vi "Teleop.vi"(10 "Match Info":T1={"Autonomous Elapsed Seconds"=0.0, "TeleOp Elapsed Seconds"=0.0, "Disabled Elapsed Seconds"=0.0, "Visited Autonomous"=FALSE, "Visited TeleOp"=FALSE, "Visited Disabled"=FALSE, "Autonomous Settings"={"Autonomous Style"=enum."Independent", "VI Refnum"=refnum}}, 11 "Call Context":T2) -> ()   [LabVIEW 2023]
doc: "This VI is called for each enabled TeleOp packet received from the DS. It is typically used to read from joysticks and other inputs and update I/O or setpoints for timed control loops. It should complete and return within 20 milliseconds or risk missing DS packets."
uses:
  <vilib>/Rock Robotics/WPI/DriverStation/WPI_DriverStationDerivedRobotMode.ctl
  <vilib>/Rock Robotics/WPI/DriverStation/WPI_DriverStationMatch Info.ctl
  <vilib>/Rock Robotics/WPI/Utilities/WPI_GetSetVariantRefNum.vi
  <vilib>/Rock Robotics/Network Tables/NT Write Boolean Array.vi
  <vilib>/Rock Robotics/Network Tables/NT Write Numeric Array.vi
  <vilib>/Rock Robotics/Network Tables/NT Read Number.vi
  MHZLib/Variables and Definitions/Robot Global Data.vi
  <vilib>/Rock Robotics/Network Tables/NT Write Boolean.vi
panel:
  out "Lift dband":dbl
  in  "Lift Lock":bool=TRUE
  out "Drive dband":dbl
  out "Steer dband":dbl
  out "Sprint Mode":bool
  out "Sprint Button":bool
  out "Sprint Throttle":dbl
  out "Drive Throttle":dbl
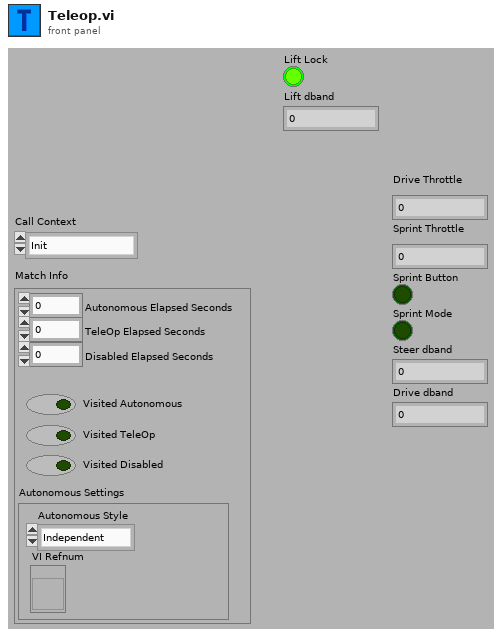
[diagram p1: front panel]
types:
  T1 = typedef "WPI_DriverStationMatch Info.ctl" = cluster{"Autonomous Elapsed Seconds":dbl, "TeleOp Elapsed Seconds":dbl, "Disabled Elapsed Seconds":dbl, "Visited Autonomous":bool, "Visited TeleOp":bool, "Visited Disabled":bool, "Autonomous Settings":cluster{"Autonomous Style":enum16{"Iterative", "Independent"}, "VI Refnum":refnum<vi>}}
  T2 = typedef "WPI_DriverStationDerivedRobotMode.ctl" = enum16{"Init", "Execute", "Stop"}
  T3 = typedef "Auto_Values.ctl" = cluster{"X Pos":dbl, "Y Pos":dbl, "Heading (Deg)":dbl, "Strafe Throttle":dbl, "Rot Throtle (Rad/s)":dbl, "Strafe Tol (Ft)":dbl, "Rotation Tol (Deg)":dbl, "Shooter Pos":enum16{"Hold", "Travel", "Speaker", "Amp"}, "Intake":enum16{"Off", "Front", "Center", "Out"}, "Auto Aim":enum16{"Off", "Aim", "Aim & Shoot"}, "Shooter Throttle":dbl, "Wait (s)":dbl, "Lift":enum16{"Off", "Up", "Down"}, "Shoot?":bool}
  T4 = typedef "WPI_JoystickDevRef.ctl" = cluster{"Device":T5}
  T5 = typedef "WPI_JoystickDeviceEnum.ctl" = enum16{"USB 0", "USB 1", "USB 2", "USB 3", "USB 4", "USB 5"}
  T6 = typedef "WPI_Joystick Info.ctl" = cluster{"Device Name":string, "HID Type":T7, "XBox Type":T8, "Axes Count":i32, "Axes Types":T9[], "Button Count":i32, "POV Count":i32}
  T7 = typedef "WPI_JoystickHID Types.ctl" = enum16{"Not HID", "HID Joystick", "HID Gamepad", "HID Driving Wheel", "HID Flightstick", "HID First Person"}
  T8 = typedef "WPI_JoystickXBox Types.ctl" = enum16{"Not XBox", "XBox Unknown", "XBox Gamepad", "XBox Wheel", "XBox Arcade Stick", "XBox Flight Stick", "XBox Dance Pad", "XBox Guitar", "XBox Drum Kit", "XBox Arcade Pad"}
  T9 = typedef "WPI_JoystickAxis Types.ctl" = enum16{"X Axis", "Y Axis", "Z Axis", "RxAxis", "RyAxis", "RzAxis", "Slider", "POV", "None", "L X Axis", "L Y Axis", "L Trigger", "R Trigger", "R X Axis", "R Y Axis"}
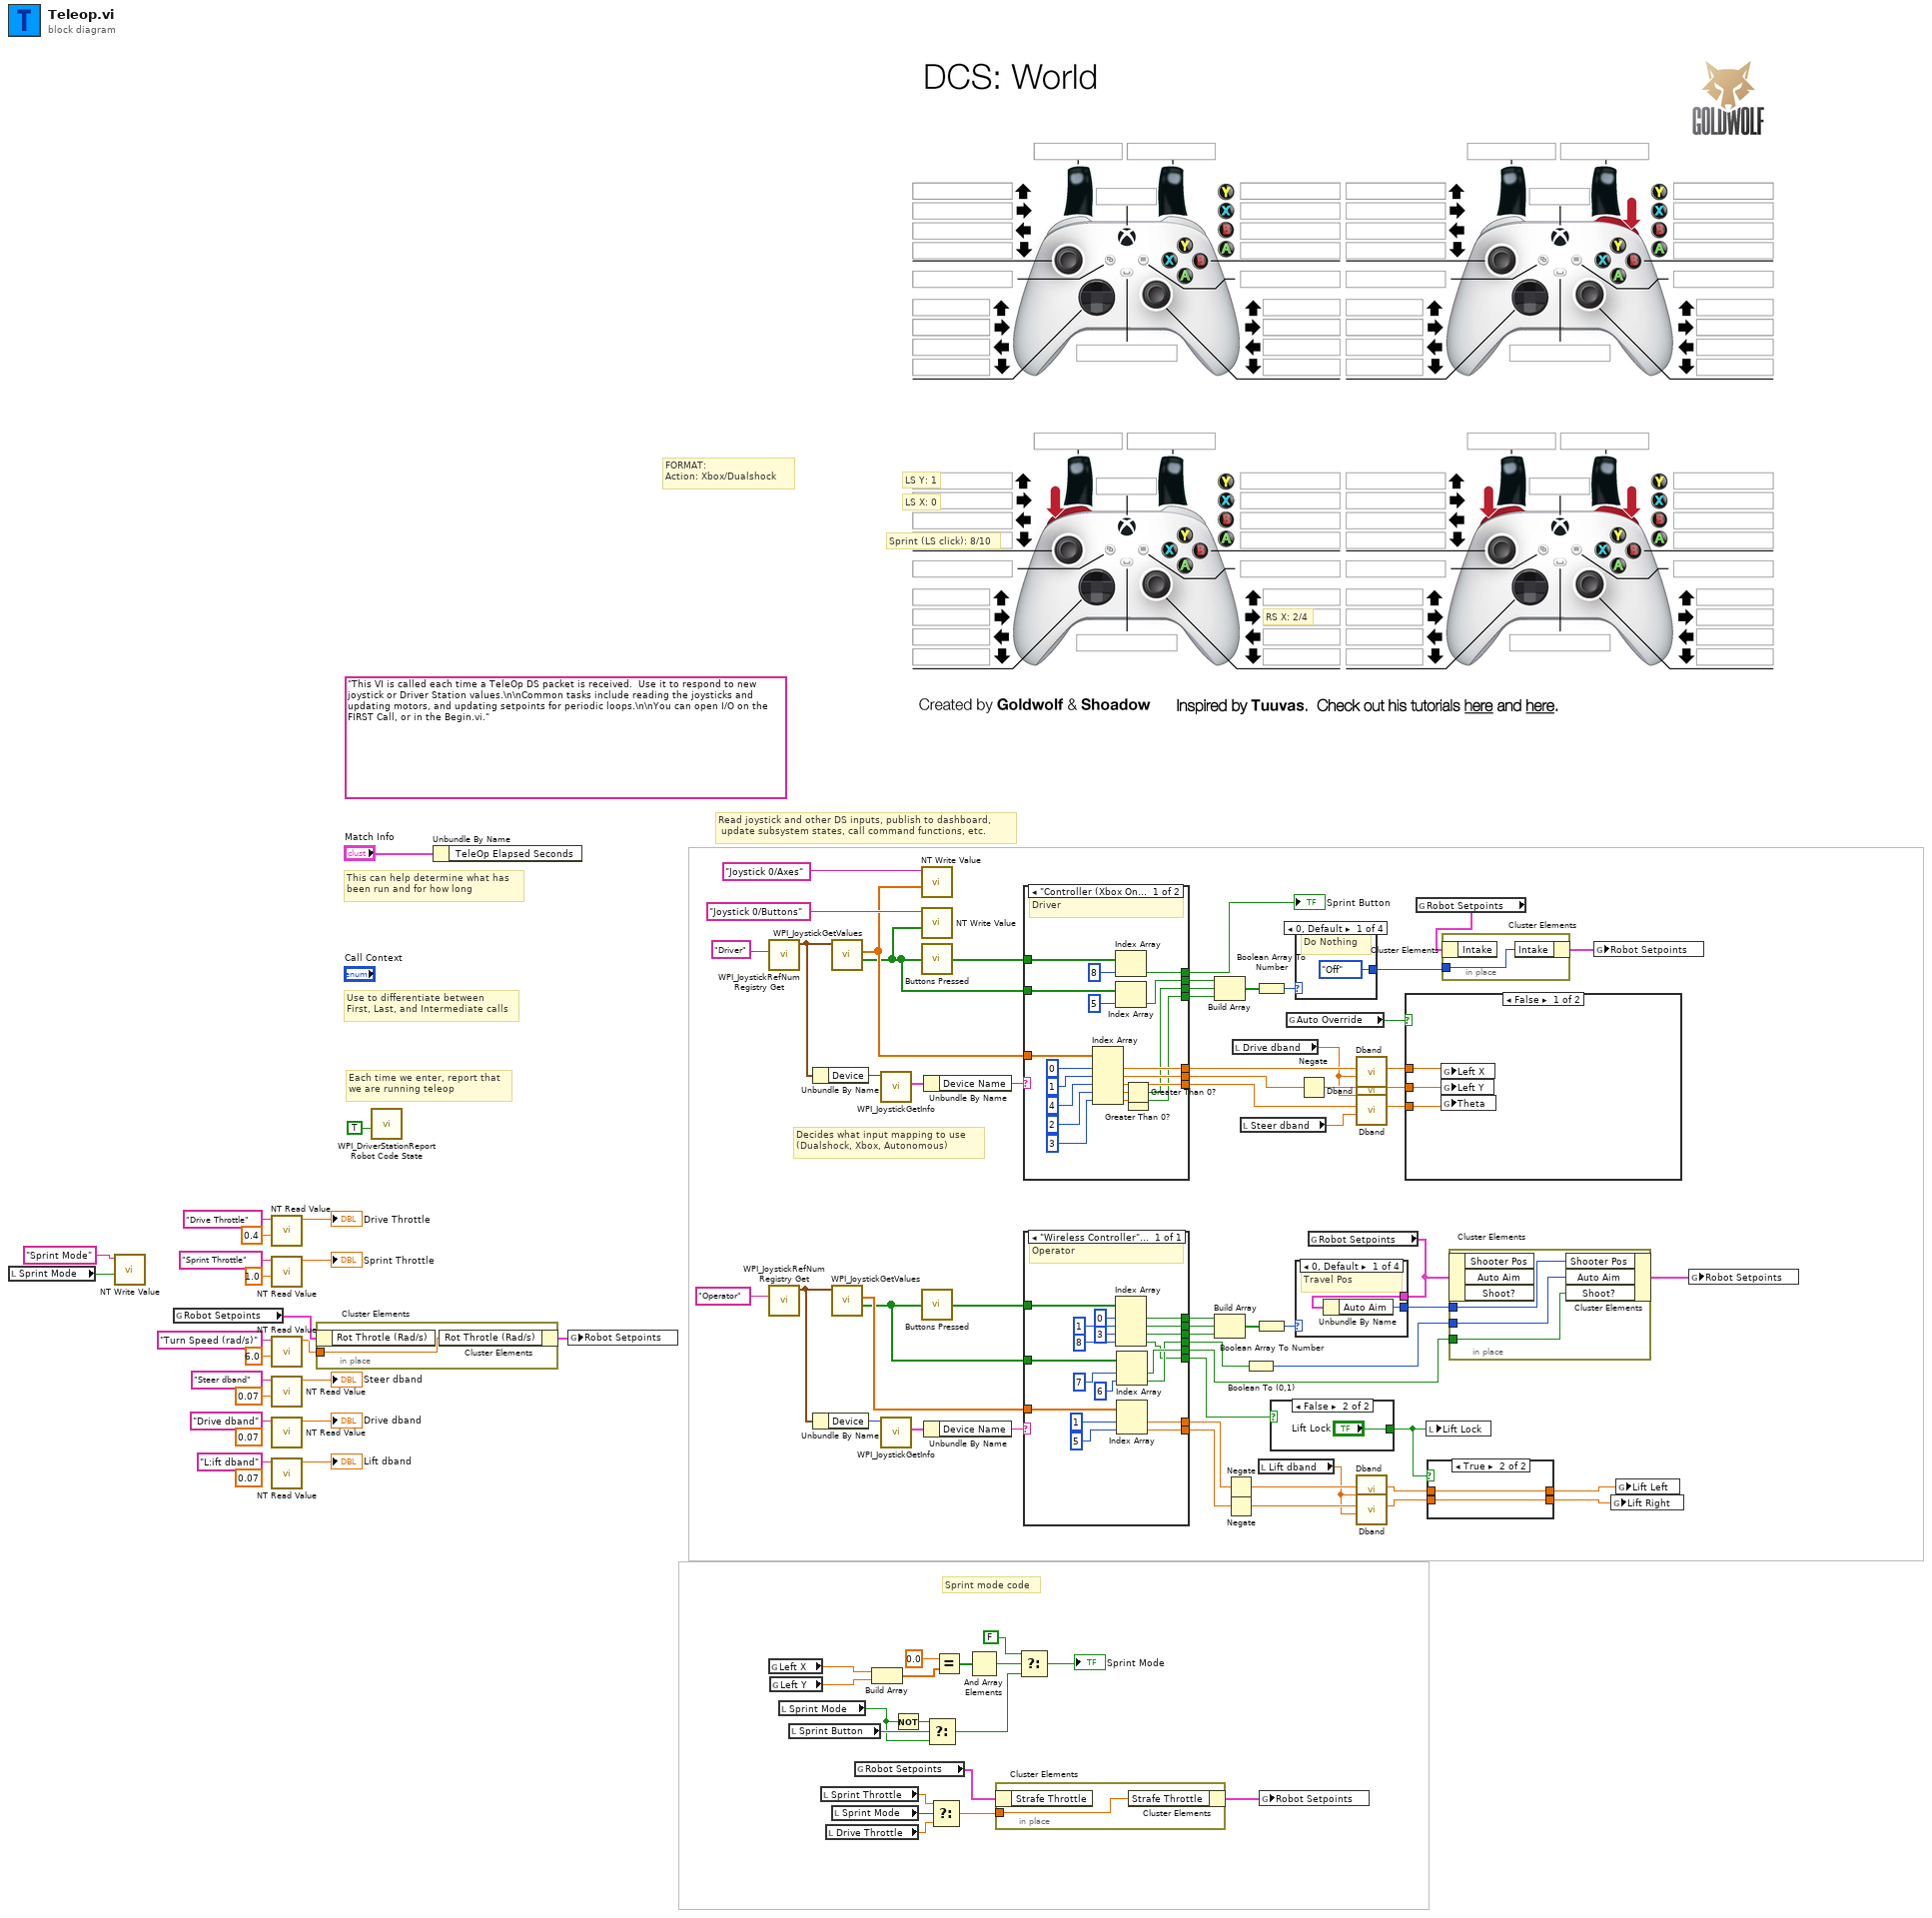
[diagram p0: block diagram]
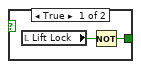
[diagram p2: hidden frame]
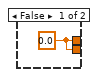
[diagram p3: hidden frame]
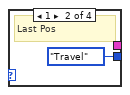
[diagram p4: hidden frame]
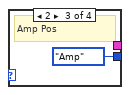
[diagram p5: hidden frame]
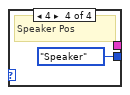
[diagram p6: hidden frame]
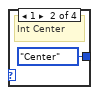
[diagram p7: hidden frame]
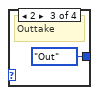
[diagram p8: hidden frame]
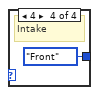
[diagram p9: hidden frame]
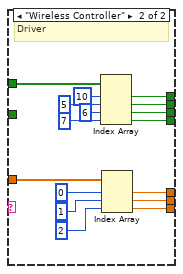
[diagram p11: hidden frame]
diagram:
  (unwired) 0.07 ("default value")
  (unwired) 0.07 ("default value")
  (unwired) "This VI is called each time a TeleOp DS packet is received.  Use it to respond to new joystick or Driver Station values.\n\nCommon tasks include reading the joysticks and updating motors, and updating setpoints for periodic loops.\n\nYou can open I/O on the FIRST Call, or in the Begin.vi."
  # "Sprint mode code"
  # "RS X: 2/4"
  # "LS X: 0"
  # "LS Y: 1"
  # "FORMAT:\nAction: Xbox/Dualshock"
  # "Sprint (LS click): 8/10"
  # "Decides what input mapping to use\n(Dualshock, Xbox, Autonomous)"
  # "Read joystick and other DS inputs, publish to dashboard,\n update subsystem states, call command functions, etc."
  # "Each time we enter, report that\nwe are running teleop"
  # "Use to differentiate between\nFirst, Last, and Intermediate calls"
  # "This can help determine what has\nbeen run and for how long"
  n1 = local read "Sprint Mode"() -> (w50:bool)
  n2 = call-poly <vilib>:"NT Write Value.vi"("value"=w50, "name"="Sprint Mode") -> ()  [unwired: 9 in, 1 out]
  n3 = global read "Robot Global Data.vi" "Robot Setpoints"() -> (w5:T3)
  n4 = call-poly <vilib>:"NT Read Value.vi"("default value"=0.4, "name"="Drive Throttle") -> ("value"=→"Drive Throttle":dbl)  [unwired: 7 in, 2 out]
  n5 = call-poly <vilib>:"NT Read Value.vi"("default value"=1.0, "name"="Sprint Throttle") -> ("value"=→"Sprint Throttle":dbl)  [unwired: 7 in, 2 out]
  n6 = call-poly <vilib>:"NT Read Value.vi"("default value"=6.0, "name"="Turn Speed (rad/s)") -> ("value"=w4:dbl)  [unwired: 7 in, 2 out]
  n7 = call-poly <vilib>:"NT Read Value.vi"("default value"=0.07, "name"="Steer dband") -> ("value"=→"Steer dband":dbl)  [unwired: 7 in, 2 out]
  n8 = call-poly <vilib>:"NT Read Value.vi"("name"="Drive dband") -> ("value"=→"Drive dband":dbl)  [unwired: 8 in, 2 out]
  n9 = call-poly <vilib>:"NT Read Value.vi"("name"="L:ift dband") -> ("value"=→"Lift dband":dbl)  [unwired: 8 in, 2 out]
  n10 = in-place {
    in-place-border: w4 -> [w100]
    n11 = in-place-cluster #1(w5) -> ()  [unwired: 1 out]
    n12 = in-place-cluster #1("Rot Throtle (Rad/s)"=w100) -> (w6:T3)
  }
  n13 = call <vilib>:"WPI_DriverStationReport Robot Code State.vi"("TeleOp"=TRUE ("Autonomous")) -> ()  [unwired: 10 in, 1 out]
  n14 = Unbundle By Name("Match Info") -> ()  [unwired: 1 out]
  n15 = global write "Robot Global Data.vi" "Robot Setpoints"(w6) -> ()
  n16 = call <vilib>:"WPI_JoystickRefNum Registry Get.vi"("refnum name"="Driver") -> ("JoystickDevRef"=w53:T4)  [unwired: 1 in, 9 out]
  n17 = call <vilib>:"WPI_JoystickRefNum Registry Get.vi"("refnum name"="Operator") -> ("JoystickDevRef"=w44:T4)  [unwired: 1 in, 9 out]
  n18 = global read "Robot Global Data.vi" "Left X"() -> (w63:dbl)
  n19 = global read "Robot Global Data.vi" "Left Y"() -> (w62:dbl)
  n20 = local read "Sprint Mode"() -> (w78:bool)
  n21 = local read "Sprint Button"() -> (w79:bool)
  n22 = Unbundle By Name(w53) -> ("Device"=w85:T5)
  n23 = Unbundle By Name(w44) -> ("Device"=w47:T5)
  n24 = local read "Sprint Throttle"() -> (w55:dbl)
  n25 = local read "Drive Throttle"() -> (w54:dbl)
  n26 = call <vilib>:"WPI_JoystickGetValues.vi"("JoystickDevRef"=w53) -> ("Buttons"=w2:bool[], "Axes"=w84:dbl[])  [unwired: 6 in, 3 out]
  n27 = call <vilib>:"WPI_JoystickGetValues.vi"("JoystickDevRef"=w44) -> ("Buttons"=w3:bool[], "Axes"=w43:dbl[])  [unwired: 6 in, 3 out]
  n28 = local read "Sprint Mode"() -> (w56:bool)
  n29 = global read "Robot Global Data.vi" "Robot Setpoints"() -> (w12:T3)
  n30 = Build Array(w63, w62) -> (w60:dbl[])
  n31 = call <vilib>:"WPI_JoystickGetInfo.vi"("JoystickDevice"=w85) -> ("Joystick Info"=w86:T6)  [unwired: 9 in, 1 out]
  n32 = call <vilib>:"WPI_JoystickGetInfo.vi"("JoystickDevice"=w47) -> ("Joystick Info"=w46:T6)  [unwired: 9 in, 1 out]
  n33 = Not(x=w78) -> (.not. x?=w80:bool)
  n34 = call-poly <vilib>:"NT Write Value.vi"("value"=w84, "name"="Joystick 0/Axes" ("Name")) -> ()  [unwired: 9 in, 1 out]
  n35 = call-poly <vilib>:"NT Write Value.vi"("value"=w2, "name"="Joystick 0/Buttons" ("Name")) -> ()  [unwired: 9 in, 1 out]
  n36 = call "Buttons Pressed.vi"("Button Values"=w2) -> ("Button Presses"=w82:bool[])
  n37 = call "Buttons Pressed.vi"("Button Values"=w3) -> ("Button Presses"=w42:bool[])
  n38 = Unbundle By Name(w86) -> ("Device Name"=w83:string)
  n39 = Unbundle By Name(w46) -> ("Device Name"=w45:string)
  n40 = Select(t=w80, s=w79, f=w78) -> (s? t:f=w52:bool)
  n41 = Select(t=w55, s=w56, f=w54) -> (s? t:f=w11:dbl)
  n42 = Equal?(x=0.0, y=w60) -> (x = y?=w59:bool[])
  n43 = And Array Elements(Boolean array=w59) -> (logical AND=w58:bool)
  n44 = in-place {
    in-place-border: w11 -> [w101]
    n45 = in-place-cluster #2(w12) -> ()  [unwired: 1 out]
    n46 = in-place-cluster #2("Strafe Throttle"=w101) -> (w10:T3)
  }
  n47 = Select(t=FALSE, s=w58, f=w52) -> (s? t:f=→"Sprint Mode":bool)
  n48 = case shown="\"Controller (Xbox One For Windows)\", Default" w83 {
    tunnel: w84 -> [w117 w133]
    tunnel: w82 -> [w115 w132]
    tunnel: [w114 w130] -> w81
    tunnel: [w113 w129] -> w68
    tunnel: [w112 w128] -> w67
    tunnel: [w111 w127] -> w66
    tunnel: [w104 w125] -> w40
    tunnel: [w106 w123] -> w39
    tunnel: [w105 w124] -> w38
    tunnel: w2 -> [w102 _]
    frame "Controller (Xbox One For Windows)", Default {
      # "Driver"
      n49 = Index Array(array=w117, index #1=0 ("index"), index #2=1 ("index"), index #3=4 ("index"), index #4=2 ("index"), index #5=3 ("index")) -> (element #1=w113:dbl, element #2=w112:dbl, element #3=w111:dbl, element #4=w108:dbl, element #5=w107:dbl)
      n50 = Index Array(array=w115, index=8) -> (element=w114:bool)
      n51 = Index Array(array=w102, index=5) -> (element=w104:bool)
      n52 = Greater Than 0?(x=w108) -> (x > 0?=w106:bool)
      n53 = Greater Than 0?(x=w107) -> (x > 0?=w105:bool)
    }
    frame "Wireless Controller" {
      # "Driver"
      n54 = Index Array(array=w132, index #1=10 ("index"), index #2=5 ("index"), index #3=6 ("index"), index #4=7 ("index")) -> (element #1=w130:bool, element #2=w125:bool, element #3=w123:bool, element #4=w124:bool)
      n55 = Index Array(array=w133, index #1=0 ("index"), index #2=1 ("index"), index #3=2 ("index")) -> (element #1=w129:dbl, element #2=w128:dbl, element #3=w127:dbl)
    }
  }
  "Sprint Button" <- w81
  n56 = case shown="\"Wireless Controller\", Default" w45 {
    tunnel: w43 -> [w153]
    tunnel: w42 -> [w152]
    tunnel: [w150] -> w35
    tunnel: [w149] -> w25
    tunnel: [w148] -> w26
    tunnel: [w146] -> w34
    tunnel: [w144] -> w33
    tunnel: [w138] -> w29
    tunnel: [w139] -> w27
    tunnel: [w137] -> w22
    tunnel: w3 -> [w140]
    frame "Wireless Controller", Default {
      # "Operator"
      n57 = Index Array(array=w152, index #1=0 ("index"), index #2=1 ("index"), index #3=3 ("index"), index #4=8 ("index")) -> (element #1=w150:bool, element #2=w146:bool, element #3=w144:bool, element #4=w137:bool)
      n58 = Index Array(array=w140, index #1=7 ("index"), index #2=6 ("index")) -> (element #1=w139:bool, element #2=w138:bool)
      n59 = Index Array(array=w153, index #1=1 ("index"), index #2=5 ("index")) -> (element #1=w149:dbl, element #2=w148:dbl)
    }
  }
  n60 = Build Array(w40, w39, w38) -> (w37:bool[])
  n61 = Build Array(w35, w34, w33) -> (w32:bool[])
  n62 = Negate(x=w25) -> (-x=w20:dbl)
  n63 = Negate(x=w26) -> (-x=w19:dbl)
  n64 = local read "Drive dband"() -> (w65:dbl)
  n65 = local read "Steer dband"() -> (w64:dbl)
  n66 = Boolean To (0,1)(Boolean=w29) -> (0, 1=w28:i16)
  n67 = Boolean Array To Number(Boolean array=w37) -> (number=w36:u32)
  n68 = Boolean Array To Number(Boolean array=w32) -> (number=w31:u32)
  n69 = local read "Lift dband"() -> (w16:dbl)
  n70 = global write "Robot Global Data.vi" "Robot Setpoints"(w10) -> ()
  n71 = case shown="False" w22 {
    tunnel: [w156 "Lift Lock"] -> w21
    frame True {
      n72 = local read "Lift Lock"() -> (w157:bool)
      n73 = Not(x=w157) -> (.not. x?=w156:bool)
    }
    frame False {
    }
  }
  n74 = global read "Robot Global Data.vi" "Auto Override"() -> (w48:bool)
  n75 = case shown="0, Default" w36 {
    tunnel: [enum16{"Off", "Front", "Center", "Out"}."Off" ("Intake") enum16{"Off", "Front", "Center", "Out"}."Center" ("Intake") enum16{"Off", "Front", "Center", "Out"}."Out" ("Intake") enum16{"Off", "Front", "Center", "Out"}."Front" ("Intake")] -> w8
    frame 0, Default {
      # "Do Nothing"
    }
    frame 1 {
      # "Int Center"
    }
    frame 2 {
      # "Outtake"
    }
    frame 4 {
      # "Intake"
    }
  }
  n76 = Negate(x=w67) -> (-x=w72:dbl)
  n77 = global read "Robot Global Data.vi" "Robot Setpoints"() -> (w1:T3)
  n78 = case shown="0, Default" w31 {
    tunnel: [w163 enum16{"Hold", "Travel", "Speaker", "Amp"}."Travel" ("Shooter Pos") enum16{"Hold", "Travel", "Speaker", "Amp"}."Amp" ("Shooter Pos") enum16{"Hold", "Travel", "Speaker", "Amp"}."Speaker" ("Shooter Pos")] -> w30
    tunnel: w1 -> [w164 _ _ _]
    frame 0, Default {
      # "Travel Pos"
      n79 = Unbundle By Name(w164) -> ("Auto Aim"=w163:enum16{"Off", "Aim", "Aim & Shoot"})
    }
    frame 1 {
      # "Last Pos"
    }
    frame 2 {
      # "Amp Pos"
    }
    frame 4 {
      # "Speaker Pos"
    }
  }
  n80 = call "Dband.vi"("dband"=w65, "Numeric"=w68) -> ("Fixed"=w69:dbl)  [unwired: 9 in]
  n81 = call "Dband.vi"("dband"=w65, "Numeric"=w72) -> ("Fixed"=w70:dbl)  [unwired: 9 in]
  n82 = call "Dband.vi"("dband"=w64, "Numeric"=w66) -> ("Fixed"=w71:dbl)  [unwired: 9 in]
  n83 = call "Dband.vi"("dband"=w16, "Numeric"=w20) -> ("Fixed"=w15:dbl)  [unwired: 9 in]
  n84 = call "Dband.vi"("dband"=w16, "Numeric"=w19) -> ("Fixed"=w14:dbl)  [unwired: 9 in]
  n85 = case shown="False" w48 {
    tunnel: w71 -> [w168 _]
    tunnel: w70 -> [w170 _]
    tunnel: w69 -> [w169 _]
    frame False {
      n86 = global write "Robot Global Data.vi" "Left X"(w169) -> ()
      n87 = global write "Robot Global Data.vi" "Left Y"(w170) -> ()
      n88 = global write "Robot Global Data.vi" "Theta"(w168) -> ()
    }
    frame True {
    }
  }
  n89 = global read "Robot Global Data.vi" "Robot Setpoints"() -> (w9:T3)
  n90 = local write "Lift Lock"(w21) -> ()
  n91 = case shown="True" w21 {
    tunnel: w14 -> [_ w173]
    tunnel: [w171 w173] -> w23
    tunnel: w15 -> [_ w172]
    tunnel: [w171 w172] -> w24
    frame False {
      w171 = 0.0 ("upper limit")
    }
    frame True {
    }
  }
  n92 = in-place {
    in-place-border: w8 -> [w174]
    n93 = in-place-cluster #3(w9) -> ()  [unwired: 1 out]
    n94 = in-place-cluster #3("Intake"=w174) -> (w7:T3)
  }
  n95 = in-place {
    in-place-border: w30 -> [w177]
    in-place-border: w28 -> [w176]
    in-place-border: w27 -> [w175]
    n96 = in-place-cluster #4(w1) -> ()  [unwired: 3 out]
    n97 = in-place-cluster #4("Shooter Pos"=w177, "Auto Aim"=w176, "Shoot?"=w175) -> (w13:T3)
  }
  n98 = global write "Robot Global Data.vi" "Robot Setpoints"(w7) -> ()
  n99 = global write "Robot Global Data.vi" "Lift Right"(w23) -> ()
  n100 = global write "Robot Global Data.vi" "Lift Left"(w24) -> ()
  n101 = global write "Robot Global Data.vi" "Robot Setpoints"(w13) -> ()
